vi "FIR Window Calculator.vi"() -> ()   [LabVIEW 2017]
uses:
  <vilib>/Analysis/3filter.llb/Filter Passband Type.ctl
  <vilib>/Analysis/4window.llb/windowTd.ctl
  <vilib>/Analysis/3filter.llb/FIR Windowed Filter (DBL).vi
  <vilib>/Analysis/NI_AALBase.lvlib
  <vilib>/measure/NI_MAPro.lvlib
  <vilib>/Analysis/NI_AALPro.lvlib
panel:
  out "Saving Data":bool
  out "Filtered FIR":dbl[](array[numeric])
  out "Input":waveform(dbl)(graph)
  in  "?":bool
  out "Output":dbl[](graph)
  in  "window":T1 items=["Rectangle"=0, "Hanning"=1, "Hamming"=2, "Blackman-Harris"=3, "Exact Blackman"=4, "Blackman"=5, "Flat Top"=6, "4 Term B-Harris "=7, "7 Term B-Harris"=8, "Low Sidelobe"=9, "Blackman Nuttall"=11, "Triangle"=30, "Bartlett-Hanning"=31, "Bohman"=32, "Parzen"=33, "Welch"=34, "Kaiser"=60, "Dolph-Chebyshev"=61, "Gaussian"=62]
  in  "high cutoff freq: fh":dbl=0.45 format="%0.2f"
  in  "low cutoff freq: fl":dbl=0.125 format="%0.2f"
  in  "filter type":T2
  in  "formula":string="sin(w*t)*sin(2*pi(1)*t)"
  in  "amplitude":dbl=1.0 format="%0.2p"
  in  "frequency":dbl=10.0 format="%0.2p"
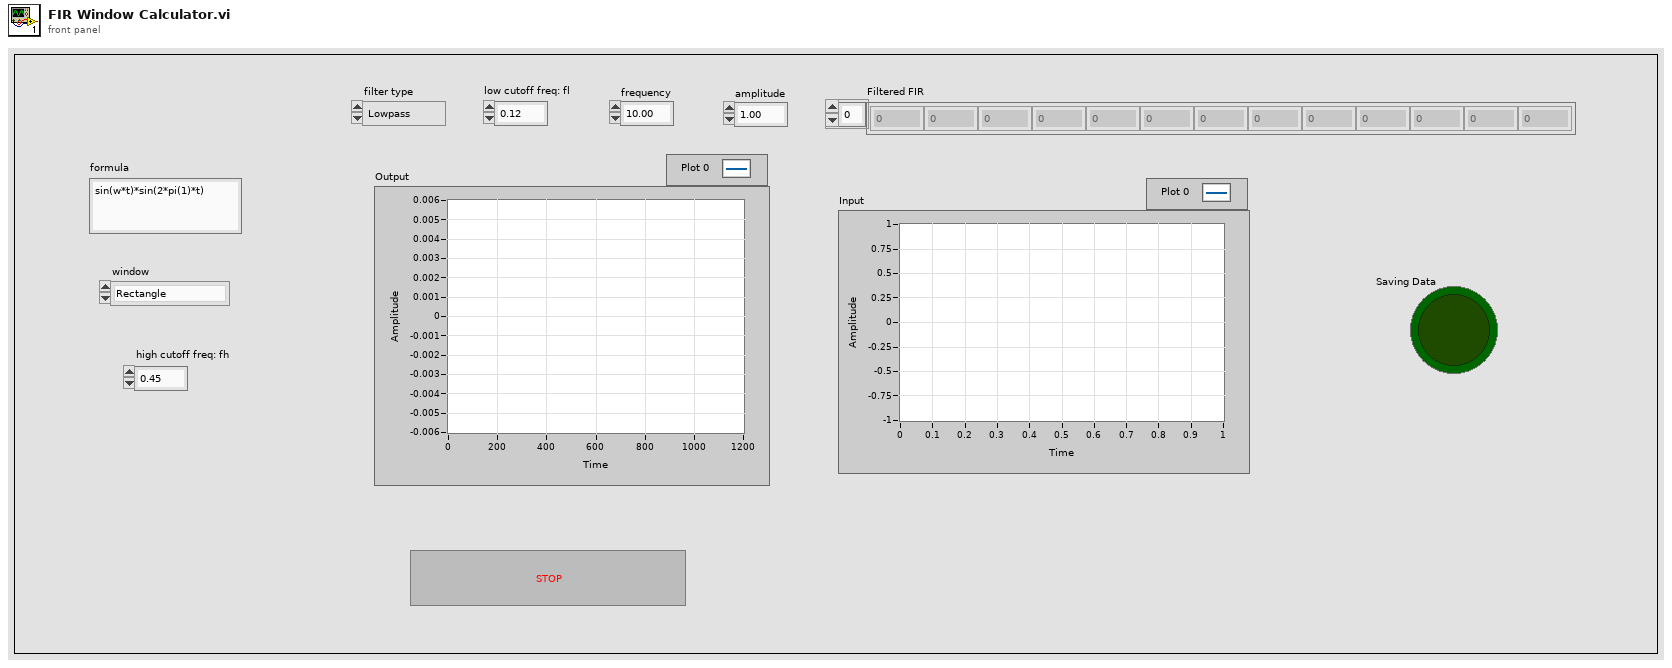
[diagram p1: front panel]
types:
  T1 = typedef "NI_AALPro.lvlib/windowTd.ctl" = u32
  T2 = typedef "NI_AALBase.lvlib/Filter Passband Type.ctl" = enum32{"Lowpass", "Highpass", "Bandpass", "Bandstop"}
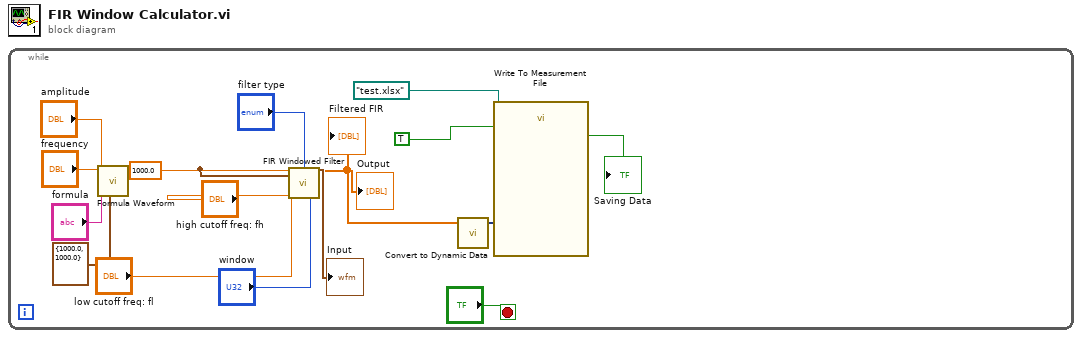
[diagram p0: block diagram]
diagram:
  n1 = while {
    stop <- "?" stop-if-true
    n2 = call <vilib>:"Formula Waveform.vi"("sampling info"=cluster{"Fs":dbl, "#s":dbl} {"Fs"=1000.0, "#s"=1000.0}, "formula"="formula", "amplitude"="amplitude", "frequency"="frequency") -> ("signal out"=w6:waveform(dbl))  [unwired: 6 in, 1 out]
    "Input" <- w6
    n3 = call-poly <vilib>:"FIR Windowed Filter.vi"("sampling freq: fs"=1000.0, "X"=w6, "filter type"="filter type", "low cutoff freq: fl"="low cutoff freq: fl", "high cutoff freq: fh"="high cutoff freq: fh", "window"="window") -> ("Filtered X"=w3:dbl[])  [unwired: 8 in, 1 out]
    "Output" <- w3
    "Filtered FIR" <- w3
    n4 = call "Convert to Dynamic Data"("Array"=w3) -> ("Dynamic Data Type"=w2:dynamicdata)  [unwired: 3 in]
    n5 = call "Write To Measurement File"("Signals"=w2, "Enable"=TRUE, "Filename"=path "test.xlsx") -> ("Saving Data"=→"Saving Data":bool)  [unwired: 14 in, 2 out]
  }
